vi "Update Da.vi"(8 "error in (no error)":errorcluster, 11 "Stand in":refnum<class "Stand.lvclass">) -> (0 "error out":errorcluster, 3 "Stand out":refnum<class "Stand.lvclass">)   [LabVIEW 2019, in "Stand.lvclass"]
uses:
  Stand.lvclass
  D:/GIT H4000/H4000/src/Device_class/Device.lvclass
  Stand.lvclass/Stand.ctl
  DI_class/DI.lvclass/DI.ctl
  DA_class/DA.lvclass/DA.ctl
  Proccess_class/Proccess.lvclass/Proccess.ctl
  Device_class/Device.lvclass/Device.ctl
  FPGA/TypeDef/AI index.ctl
  FPGA/TypeDef/DO index.ctl
  DO_class/DO.lvclass/DO.ctl
  AI_class/AI.lvclass/AI.ctl
  subvis/bool_change.vi
  DA_class/private/write_to_db.vi
  Proccess_class/GetNames.vi
  Proccess_class/GetLogger.vi
  DA_class/DA.lvclass
  D:/GIT H4000/H4000/src/Proccess_class/Proccess.lvclass
  Logger_class/WriteEvent.vi
  FPGA_API_class/FPGA API.lvclass
  DI_class/DI.lvclass
  Device_class/Device.lvclass
  AI_class/AI.lvclass
  DO_class/DO.lvclass
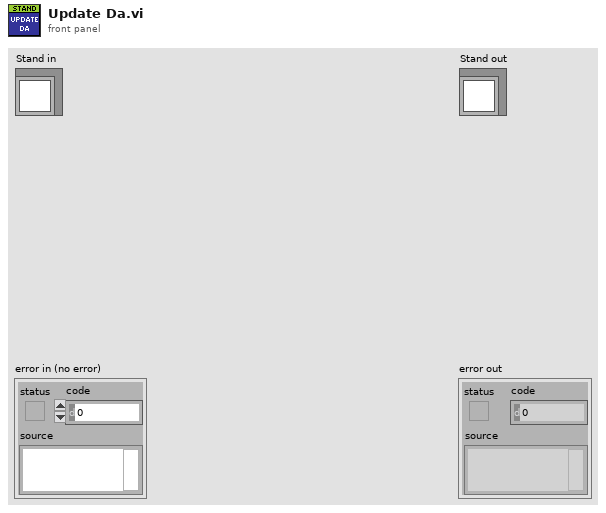
[diagram p1: front panel]
types:
  T1 = typedef "AI index.ctl" = u8
  T2 = typedef "DO index.ctl" = u8
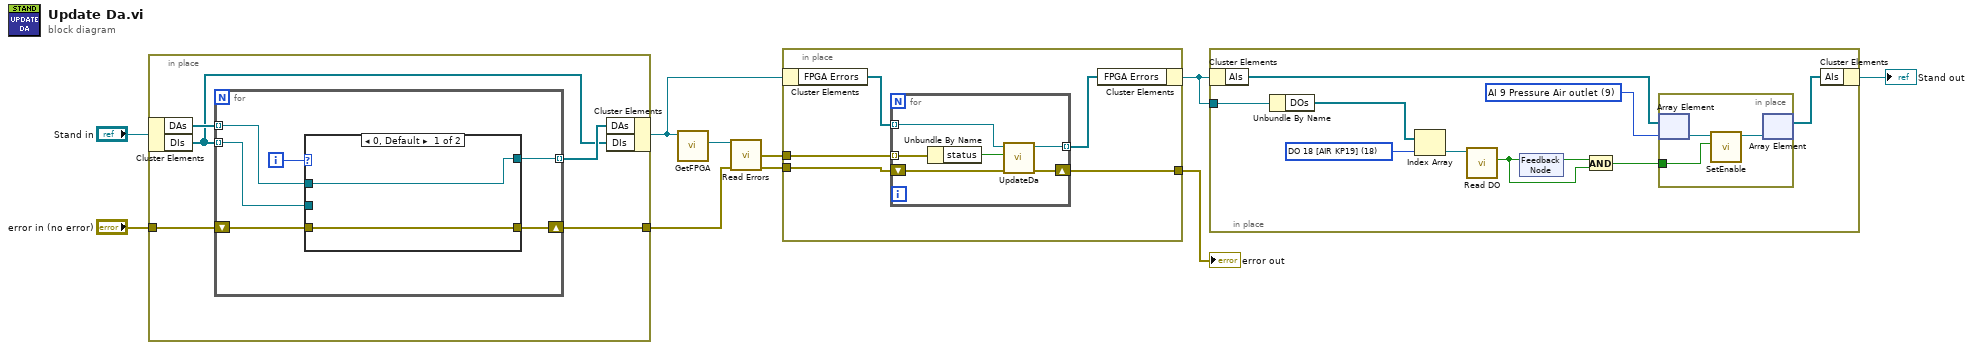
[diagram p0: block diagram]
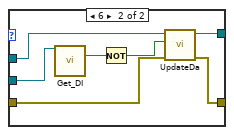
[diagram p2: hidden frame]
diagram:
  n1 = in-place {
    in-place-border: "error in (no error)" -> [w12]
    in-place-border: [w11] -> w8
    n2 = in-place-cluster #1("Stand in") -> ("DAs"=w15:refnum<class "DA.lvclass">[], "DIs"=w13:refnum<class "DI.lvclass">[])
    n3 = for {
      tunnel: w15 -> [w21] mode=indexing
      tunnel: [w20] -> w14 mode=indexing
      tunnel: w13 -> [w19] mode=indexing
      shift-right: [w17] -> w11
      shift-left: w12 -> [w18]
      i -> [w16]
      n4 = case shown="0, Default" w16 {
        tunnel: w21 -> [w23 w30]
        tunnel: [w23 w29] -> w20
        tunnel: w19 -> [_ w28]
        tunnel: w18 -> [w22 w25]
        tunnel: [w22 w24] -> w17
        frame 0, Default {
        }
        frame 6 {
          n5 = call "Get_DI.vi"("reference in"=w28) -> ("DI"=w27:bool)  [unwired: 14 in]
          n6 = Not(x=w27) -> (.not. x?=w26:bool)
          n7 = call "UpdateDa.vi"("error in (no error)"=w25, "RAW"=w26, "Sig_DA in"=w30) -> ("error out"=w24:errorcluster, "Sig_DA out"=w29:refnum<class "DA.lvclass">)  [unwired: 6 in, 1 out]
        }
      }
    }
    n8 = in-place-cluster #1("DAs"=w14, "DIs"=w13) -> (w7:refnum<class "Stand.lvclass">)
  }
  n9 = call "GetFPGA.vi"("Device in"=w7) -> ("FPGA API.lvclass"=w6:refnum<class "FPGA API.lvclass">)  [unwired: 10 in]
  n10 = call-dynamic "Read Errors.vi"("FPGA API in"=w6, "error in (no error)"=w8) -> ("Errors"=w5:errorcluster[], "error out"=w4:errorcluster)  [unwired: 11 in, 1 out]
  n11 = in-place {
    in-place-border: w4 -> [w33]
    in-place-border: w5 -> [w32]
    in-place-border: [w31] -> w2
    n12 = in-place-cluster #2(w7) -> ("FPGA Errors"=w35:refnum<class "DA.lvclass">[])
    n13 = for {
      tunnel: w35 -> [w41] mode=indexing
      tunnel: [w40] -> w34 mode=indexing
      shift-right: [w38] -> w31
      shift-left: w33 -> [w39]
      tunnel: w32 -> [w37] mode=indexing
      n14 = Unbundle By Name(w37) -> ("status"=w36:bool)
      n15 = call "UpdateDa.vi"("error in (no error)"=w39, "RAW"=w36, "Sig_DA in"=w41) -> ("error out"=w38:errorcluster, "Sig_DA out"=w40:refnum<class "DA.lvclass">)  [unwired: 6 in, 1 out]
    }
    n16 = in-place-cluster #2("FPGA Errors"=w34) -> (w3:refnum<class "Stand.lvclass">)
  }
  "error out" <- w2
  n17 = in-place {
    in-place-border: w3 -> [w49]
    w45 = T1 9 items=["AI 0 Cooling Station Level", "AI 1 Cooling Station Temp", "AI 2 Oil Supply Level", "AI 3 Oil Supply Temp", "AI 4 ", "AI 5 Pressure Haskel", "AI 6 Pressure DUT", "AI 7 Pressure Chamber", "AI 8 Pressure Air inlet", "AI 9 Pressure Air outlet", "AI 10 Pressure Messure Line"] ("AI index")
    w47 = T2 18 items=["DO 0 [KP1] [M12]", "DO 1 [ON KP2] [M21]", "DO 2 [ON KP3] [M24]", "DO 3 [WATER Y18.1 [DO3]]", "DO 4 [WATER Y18.2 [DO4]]", "DO 5 [KP6 Y29.1 33.7]", "DO 6 [KP7 Y29.2 33.8]", "DO 7 [KP8 Y29.3 33.9]", "DO 8 [KP9 Y29.4  33.12]", "DO 9 [KP10 Y29.5 33.1]", "DO 10 [KP11 Y29.6 33.2]", "DO 11 [KP12 Y29.7  33.13]", "DO 12 [KP13 Y29.8  33.11]", "DO 13 [KP14 Y29.9 33.10]", "DO 14 [KP15 Y29.10  33.6]", "DO 15 [KP16 Y29.11  33.5]", "DO 16 [KP17 Y29.12  33.4]", "DO 17 [KP18 Y29.13 33.3]", "DO 18 [AIR KP19]", "DO 19 [STEP DRIVE EN KP20]", "DO 20 [KP21 Y44.1 OPEN]", "DO 21 [ KP22 Y44.1 CLOSE]", "DO 22 [ KP23 Y44.2 OPEN]", "DO 23", "DO 24 [STEP DRIVE 1]", "DO 25 [STEP DRIVE 2]"] ("DO index")
    n18 = in-place-cluster #3(w3) -> ("AIs"=w51:refnum<class "AI.lvclass">[])
    n19 = Unbundle By Name(w49) -> ("DOs"=w48:refnum<class "DO.lvclass">[])
    n20 = Index Array(array=w48, index=w47) -> (element=w46:refnum<class "DO.lvclass">)
    n21 = call "Read DO.vi"("DO in"=w46) -> ("DO"=w42:bool)  [unwired: 9 in, 1 out]
    n22 = feedback-in #4(w42) -> ()
    n23 = feedback #4() -> (w44:bool)  [unwired: 1 in]
    n24 = And(x=w44, y=w42) -> (x .and. y?=w43:bool)
    n25 = in-place {
      in-place-border: w43 -> [w52]
      n26 = in-place-array #5(w51, w45) -> (w54:refnum<class "AI.lvclass">)
      n27 = call "SetEnable.vi"("Enable"=w52, "AI in"=w54) -> ("AI out"=w53:refnum<class "AI.lvclass">)  [unwired: 9 in]
      n28 = in-place-array #5(w53) -> (w50:refnum<class "AI.lvclass">[])  [unwired: 1 out]
    }
    n29 = in-place-cluster #3("AIs"=w50) -> (→"Stand out":refnum<class "Stand.lvclass">)
  }
